vi "Exit With Empty Queue Check.vi"(7 "Queue":refnum<queue>, 9 "Timeout (5s)":dbl=5.0, 11 "Stop":bool) -> (1 "Since Exiting (s)":dbl format="%.2f", 3 "Exit":bool)   [LabVIEW 2017, in "Communicable State Machine.lvlib"]
doc: "This VI is used for global log monitoring loops utilizing the global log queue, such as `template/CSM - Global Log Queue Monitoring Loop.vi` or the background thread of the CSM File Logger.\n\nTypically, the exit condition for these global log monitoring loops is met when the program exits. At this time, logs in the queue may not have been fully processed. Use this VI to allow a period of **Timeout (5s)** to process logs in the queue after the **Stop** signal arrives. The **Exit** signal is set to TRUE to exit the loop, only when the number of logs in the queue is empty or the timeout occurs.\n\n-- <b>Controls</b> --\n\n- <b>Queue</b>: Queue resource, such as the global log queue.\n- <b>Stop</b>: Input stop signal. When this signal is TRUE, it starts checking if the queue is empty.\n\n-- <b>Controls</b> --\n\n- <b>Timeout (5s)</b>: Timeout duration. Default is 5 s.\n- <b>Exit</b>: Real exit signal. **Exit** returns TRUE when the queue is empty or timeout occurs.\n- <b>Since Exiting (s)</b>: Time elapsed since exiting started, in seconds."
uses:
  Communicable State Machine.lvlib
  _Support/Typedef/_CSM_GlobalLog_MSG.ctl
  _Support/Typedef/_CSM_Response Source Message.ctl
  _Support/Typedef/_CSM_GlobalLog_MSG_TYPE.ctl
  _Shared/CSM Shared.lvlib
panel:
  out "# elements in queue":i32
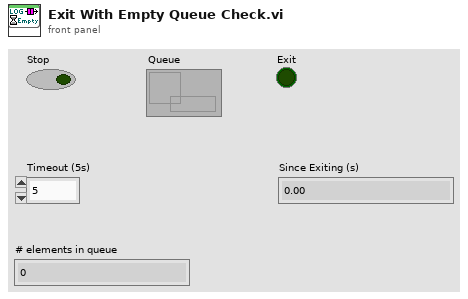
[diagram p1: front panel]
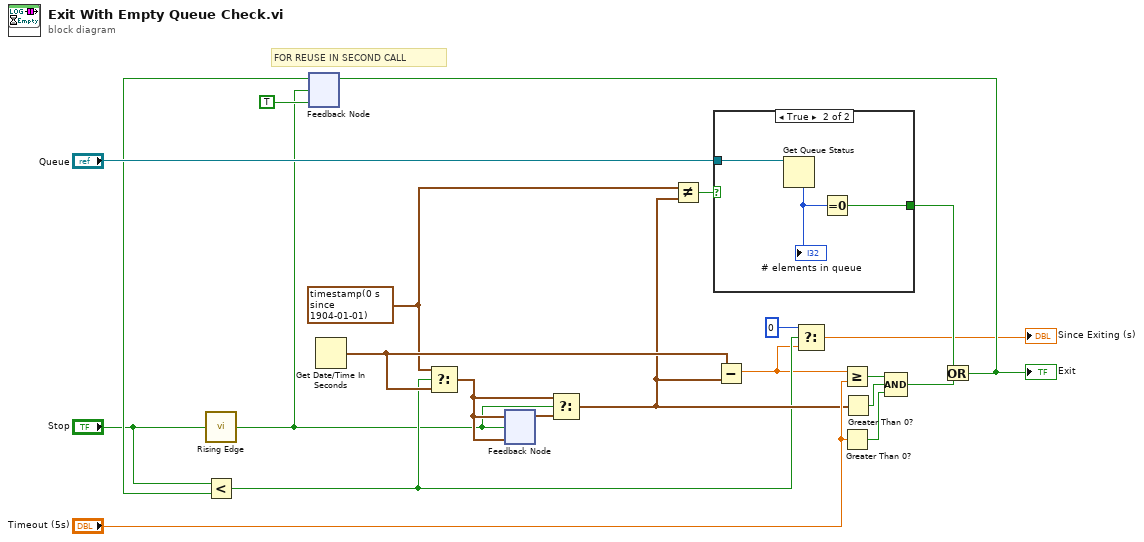
[diagram p0: block diagram]
diagram:
  w3 = timestamp(0 s since 1904-01-01)
  # "FOR REUSE IN SECOND CALL"
  n1 = call "Rising Edge.vi"("Signal"="Stop") -> ("Rising Edge"=w1:bool)
  n2 = feedback #1(TRUE) -> (w14:bool)
  n3 = Less?(x="Stop", y=w14) -> (x < y?=w6:bool)
  n4 = Get Date/Time In Seconds() -> (seconds since 1Jan1904=w12:timestamp)
  n5 = Select(t=w3, s=w6, f=w12) -> (s? t:f=w9:timestamp)
  n6 = feedback #2(w9) -> (w10:timestamp)
  n7 = feedback-in #2(w9, w1) -> ()
  n8 = Select(t=w9, s=w1, f=w10) -> (s? t:f=w8:timestamp)
  n9 = Not Equal?(x=w3, y=w8) -> (x != y?=w13:bool)
  n10 = case shown="True" w13 {
    tunnel: [_ w24] -> w18
    tunnel: "Queue" -> [_ w23]
    frame False {
    }
    frame True {
      n11 = Get Queue Status(queue=w23) -> (# elements in queue=w25:i32)  [unwired: 2 in, 7 out]
      "# elements in queue" <- w25
      n12 = Equal To 0?(x=w25) -> (x = 0?=w24:bool)
    }
  }
  n13 = Subtract(x=w12, y=w8) -> (x-y=w5:dbl)
  n14 = Select(t=u32 0 ("f"), s=w6, f=w5) -> (s? t:f=→"Since Exiting (s)":dbl)
  n15 = Greater Or Equal?(x=w5, y="Timeout (5s)") -> (x >= y?=w21:bool)
  n16 = Greater Than 0?(x="Timeout (5s)") -> (x > 0?=w20:bool)
  n17 = Greater Than 0?(x=w8) -> (x > 0?=w11:bool)
  n18 = Compound Arithmetic op=AND(w21, w11, w20) -> (w19:bool)
  n19 = Or(x=w18, y=w19) -> (x .or. y?=w16:bool)
  "Exit" <- w16
  n20 = feedback-in #1(w16, w1) -> ()
